vi "robust network stream trial.vi"() -> ()   [LabVIEW 2018]
panel:
  out "recieved data":sgl[][](array[numeric])
  out "data points received":u32
  out "timed out":bool
  in  "STOP":bool
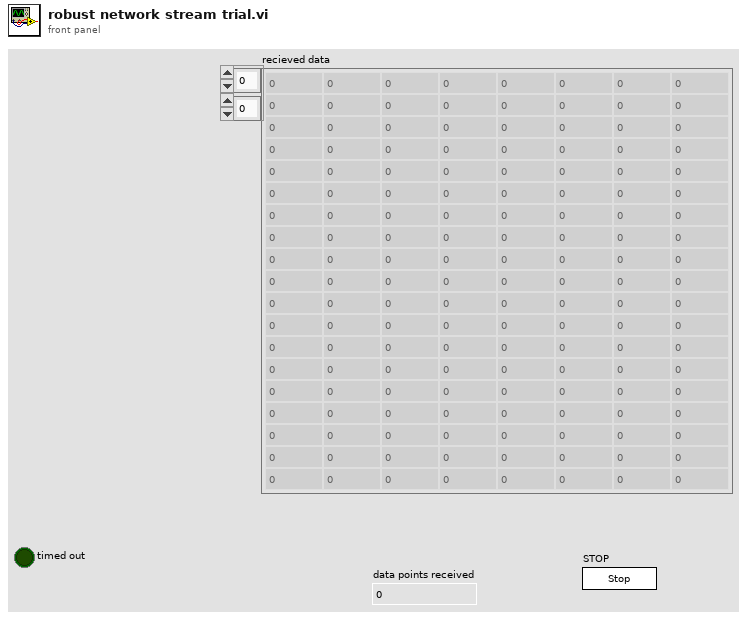
[diagram p1: front panel]
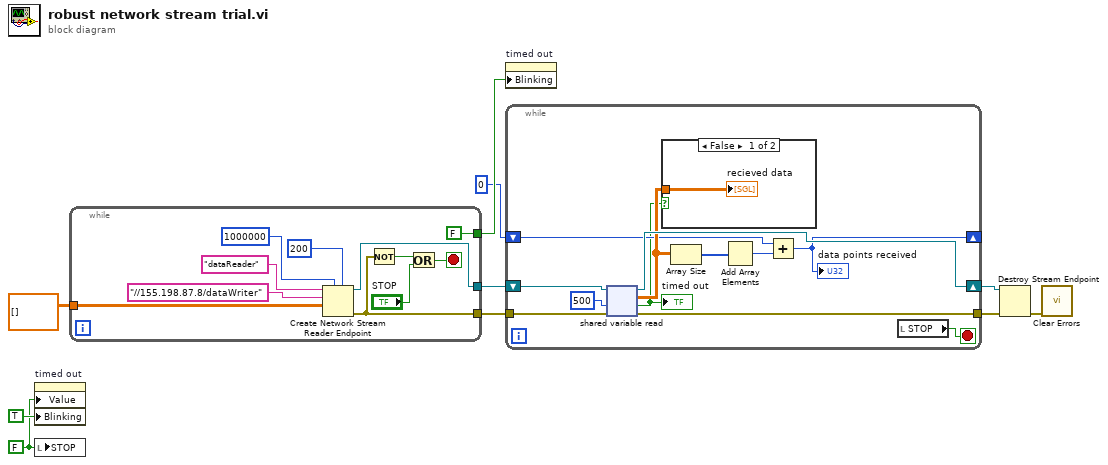
[diagram p0: block diagram]
diagram:
  w3 = FALSE ("timed out")
  n1 = property on="timed out" class="Bool (strict)"("Value"=w3, "Blinking"=TRUE) -> ()  [unwired: 2 in, 2 out]
  n2 = local write "STOP"(w3) -> ()
  n3 = while {
    tunnel: [w19] -> w8
    tunnel: [w15] -> w7
    tunnel: [FALSE ("Blinking")] -> w6
    tunnel: sgl[][] [] -> [w11]
    stop <- w14 stop-if-true
    n4 = Create Network Stream Reader Endpoint(5:200 ("timeout in ms (-1)"), 7:1000000 ("reader buffer size"), 9:w11, 10:"//155.198.87.8/dataWriter" ("writer url"), 11:"dataReader" ("reader name")) -> (0:w15:errorcluster, 3:w19:refnum<k21>)  [unwired: 2 in]
    n5 = Not(x=w15) -> (.not. x?=w16:bool)
    n6 = Or(x=w16, y="STOP") -> (x .or. y?=w14:bool)
  }
  n7 = property on="timed out" class="Bool (strict)"("Blinking"=w6) -> ()  [unwired: 2 in, 2 out]
  n8 = while {
    tunnel: w7 -> [w31]
    shift-right: [w30] -> w9
    shift-left: w8 -> [w32]
    tunnel: [w29] -> w10
    shift-right: [w25] -> _
    shift-left: u32 0 ("size(s)") -> [w26]
    stop <- w33 stop-if-true
    n9 = shared-variable-read(w32, w31, 500 ("timeout ms (-1)")) -> (w30:refnum<k21>, w29:errorcluster, w24:bool, w27:sgl[][])
    "timed out" <- w24
    n10 = case shown="False" w24 {
      tunnel: w27 -> [w34 _]
      frame False {
        "recieved data" <- w34
      }
      frame True {
      }
    }
    n11 = Array Size(array=w27) -> (size(s)=w23:i32[])
    n12 = Add Array Elements(numeric array=w23) -> (sum=w22:i32)
    n13 = Add(x=w26, y=w22) -> (x+y=w25:u32)
    "data points received" <- w25
    n14 = local read "STOP"() -> (w33:bool)
  }
  n15 = Destroy Stream Endpoint(8:w10, 11:w9) -> (0:w5:errorcluster)
  n16 = call <vilib>:"Clear Errors.vi"("error in (no error)"=w5) -> ()  [unwired: 5 in, 2 out]
